vi "PLC.IO.vi"(7 "Idx":i32, 8 "error in":errorcluster, 10 "DbRun":bool, 11 "Data_in":T1={"Status"={"Idx"=0, "ConnRef"=0, "State"=enum."Off", "LiveBitTimer"=timestamp(0 s since 1904-01-01)}, "Sets"={"Enable"=FALSE, "IP"="", "Rack"=0, "Slot"=0, "LifeBitTimer_s"=0.0, "DataBlockAddr_PCStatus"=0, "DataBlockAddr_PLCStatus"=1, "DataBlockAddr_PLCNewData"=[], "DataBlockSize_PLCNewData"=[], "DataBlockAddr_PLCChangeOver"=[], "DataBlockSize_PLCChangeOver"=[], "DataBlockAddr_PCChangeOver"=[], "DataBlockAddr_PLCCheckStatus"=[], "DataBlockSize_PLCCheckStatus"=[], "DataBlockAddr_PCCheckStatus"=[], "System"=""}, "PCstatus"={"General"={"LifeBit"=FALSE, "DbRun"=FALSE}, "Stations"=[]}, "PLCstatus"={"General"={"LifeBit"=FALSE}, "Stations"=[]}}) -> (0 "error out":errorcluster, 3 "Data_out":T1={"Status"={"Idx"=0, "ConnRef"=0, "State"=enum."Off", "LiveBitTimer"=timestamp(0 s since 1904-01-01)}, "Sets"={"Enable"=FALSE, "IP"="", "Rack"=0, "Slot"=0, "LifeBitTimer_s"=0.0, "DataBlockAddr_PCStatus"=0, "DataBlockAddr_PLCStatus"=1, "DataBlockAddr_PLCNewData"=[], "DataBlockSize_PLCNewData"=[], "DataBlockAddr_PLCChangeOver"=[], "DataBlockSize_PLCChangeOver"=[], "DataBlockAddr_PCChangeOver"=[], "DataBlockAddr_PLCCheckStatus"=[], "DataBlockSize_PLCCheckStatus"=[], "DataBlockAddr_PCCheckStatus"=[], "System"=""}, "PCstatus"={"General"={"LifeBit"=FALSE, "DbRun"=FALSE}, "Stations"=[]}, "PLCstatus"={"General"={"LifeBit"=FALSE}, "Stations"=[]}})   [LabVIEW 2016]
doc: "Read data block from PLC to PC and write data block from PC to PLC. Control live bit of PC\n\nWabco 2017 All right reserved\nAuthor: maciej.szupienko@wabco-auto.com"
uses:
  PLC.Data.ctl
  PLC.Data.Status.ctl
  PLC.State.ctl
  PLC.Data.Sets.ctl
  LowLevel/PLC.DataBlock.PCstatus.ctl
  LowLevel/PLC.DataBlock.PCstatus.General.ctl
  LowLevel/PLC.DataBlock.PCstatus.Station.ctl
  LowLevel/PLC.DataBlock.PLCstatus.ctl
  LowLevel/PLC.DataBlock.PLCstatus.General.ctl
  LowLevel/PLC.DataBlock.PLCstatus.Station.ctl
  tools/EventLog/EventLog.EventSource.ctl
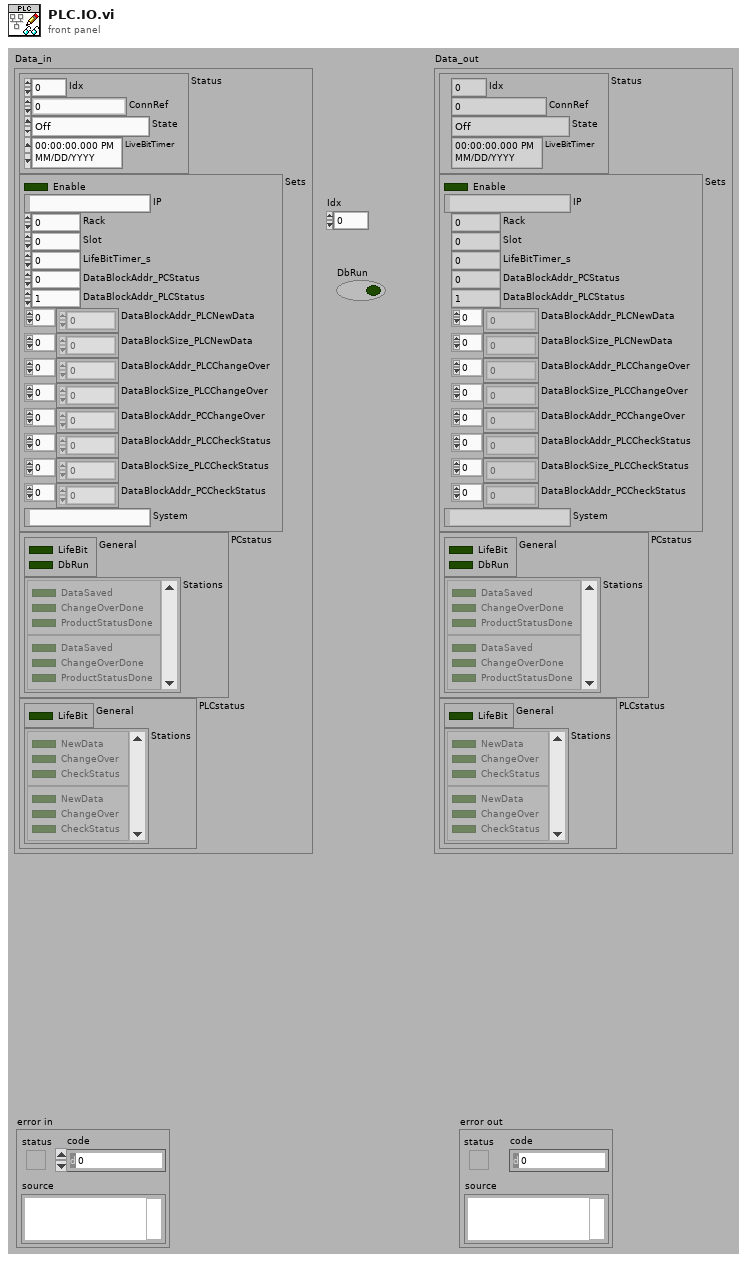
[diagram p1: front panel]
types:
  T1 = typedef "PLC.Data.ctl" = cluster{"Status":T2, "Sets":T4, "PCstatus":T5, "PLCstatus":T8}
  T2 = typedef "PLC.Data.Status.ctl" = cluster{"Idx":i32, "ConnRef":u64, "State":T3, "LiveBitTimer":timestamp}
  T3 = typedef "PLC.State.ctl" = enum32{"Off", "Error", "Idle", "Run"}
  T4 = typedef "PLC.Data.Sets.ctl" = cluster{"Enable":bool, "IP":string, "Rack":i32, "Slot":i32, "LifeBitTimer_s":dbl, "DataBlockAddr_PCStatus":i32, "DataBlockAddr_PLCStatus":i32, "DataBlockAddr_PLCNewData":i32[], "DataBlockSize_PLCNewData":i32[], "DataBlockAddr_PLCChangeOver":i32[], "DataBlockSize_PLCChangeOver":i32[], "DataBlockAddr_PCChangeOver":i32[], "DataBlockAddr_PLCCheckStatus":i32[], "DataBlockSize_PLCCheckStatus":i32[], "DataBlockAddr_PCCheckStatus":i32[], "System":string}
  T5 = typedef "PLC.DataBlock.PCstatus.ctl" = cluster{"General":T6, "Stations":T7[]}
  T6 = typedef "PLC.DataBlock.PCstatus.General.ctl" = cluster{"LifeBit":bool, "DbRun":bool}
  T7 = typedef "PLC.DataBlock.PCstatus.Station.ctl" = cluster{"DataSaved":bool, "ChangeOverDone":bool, "ProductStatusDone":bool}
  T8 = typedef "PLC.DataBlock.PLCstatus.ctl" = cluster{"General":T9, "Stations":T10[]}
  T9 = typedef "PLC.DataBlock.PLCstatus.General.ctl" = cluster{"LifeBit":bool}
  T10 = typedef "PLC.DataBlock.PLCstatus.Station.ctl" = cluster{"NewData":bool, "ChangeOver":bool, "CheckStatus":bool}
  T11 = typedef "EventLog.EventSource.ctl" = enum16{"All", "Gui", "Ref", "File", "Arch", "Seq", "CPX", "DB", "Laser", "Scan.P", "Scan.O", "PLC"}
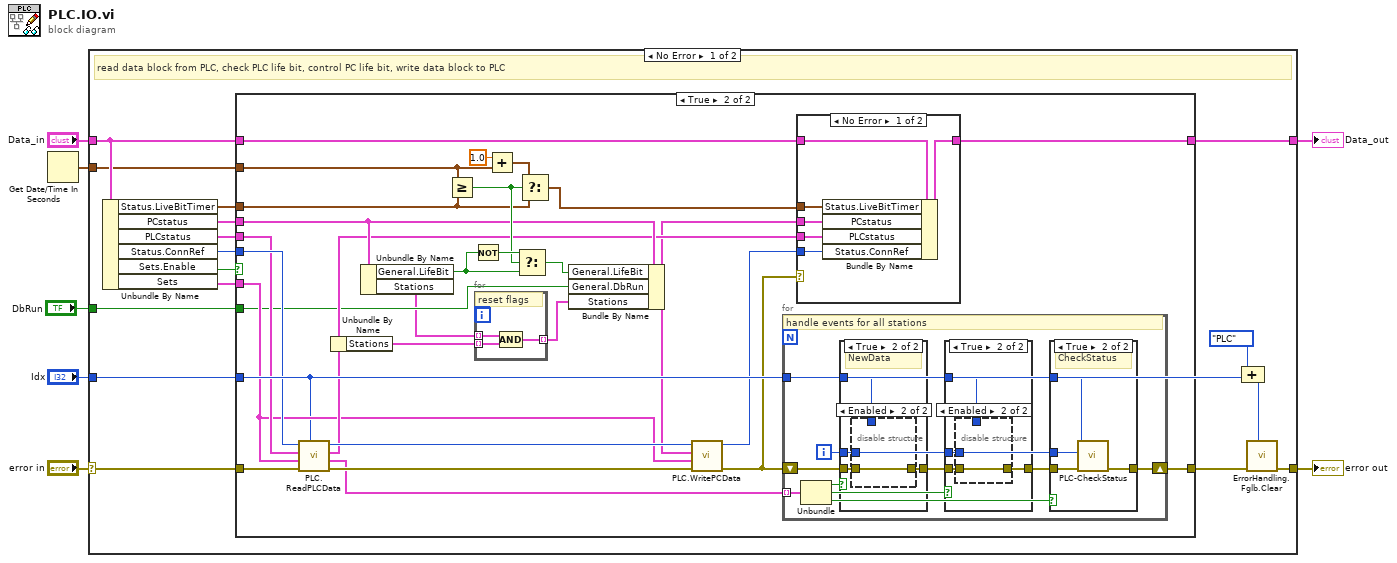
[diagram p0: block diagram]
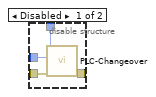
[diagram p5: hidden frame]
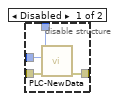
[diagram p7: hidden frame]
diagram:
  n1 = Get Date/Time In Seconds() -> (seconds since 1Jan1904=w3:timestamp)
  n2 = case shown="No Error" "error in" {
    selector: "error in" -> [w20 w101]
    tunnel: [w22 w101] -> w4
    tunnel: "Data_in" -> [w21 w100]
    tunnel: [w23 w100] -> w6
    tunnel: w3 -> [w19 _]
    tunnel: "Idx" -> [w11 _]
    tunnel: "DbRun" -> [w9 _]
    frame No Error {
      # "read data block from PLC, check PLC life bit, control PC life bit, write data block to PLC"
      n3 = Unbundle By Name(w21) -> ("Status.LiveBitTimer"=w18:timestamp, "PCstatus"=w17:T5, "PLCstatus"=w14:T8, "Status.ConnRef"=w16:u64, "Sets.Enable"=w13:bool, "Sets"=w12:T4)
      n4 = case shown="True" w13 {
        tunnel: [w25 w54] -> w23
        tunnel: w21 -> [w25 w53]
        tunnel: w20 -> [w24 w39]
        tunnel: w19 -> [_ w50]
        tunnel: w18 -> [_ w49]
        tunnel: w17 -> [_ w48]
        tunnel: w16 -> [_ w41]
        tunnel: [w24 w45] -> w15
        tunnel: w14 -> [_ w40]
        tunnel: w12 -> [_ w35]
        tunnel: w11 -> [_ w34]
        tunnel: w9 -> [_ w30]
        frame False {
        }
        frame True {
          n5 = call "PLC.ReadPLCData.vi"("Idx"=w34, "error in (no error)"=w39, "Sets"=w35, "PLCdata in"=w40, "Ref in"=w41) -> ("error out"=w36:errorcluster, "Events"=w31:T10[], "PLCdata out"=w37:T8, "Ref out"=w38:u64)  [unwired: 3 in]
          n6 = Unbundle By Name(w37) -> ("Stations"=w47:T10[])
          n7 = Unbundle By Name(w48) -> ("General.LifeBit"=w46:bool, "Stations"=w29:T7[])
          n8 = Greater Or Equal?(x=w50, y=w49) -> (x >= y?=w51:bool)
          n9 = Not(x=w46) -> (.not. x?=w52:bool)
          n10 = for {
            tunnel: w47 -> [w91] mode=indexing
            tunnel: w29 -> [w92] mode=indexing
            tunnel: [w90] -> w27 mode=indexing
            # "reset flags"
            n11 = Compound Arithmetic op=AND(w92, w91) -> (w90:T7)
          }
          n12 = Add(x=1.0 ("y"), y=w50) -> (x+y=w44:timestamp)
          n13 = Select(t=w52, s=w51, f=w46) -> (s? t:f=w26:bool)
          n14 = Select(t=w44, s=w51, f=w49) -> (s? t:f=w42:timestamp)
          n15 = Bundle By Name(cluster=w48, "General.LifeBit"=w26, "General.DbRun"=w30, "Stations"=w27) -> (w28:T5)
          n16 = call "PLC.WritePCData.vi"("error in (no error)"=w36, "Sets"=w35, "PCdata in"=w28, "Ref in"=w38) -> ("error out"=w32:errorcluster, "Ref out"=w33:u64)  [unwired: 5 in, 1 out]
          n17 = for {
            tunnel: w34 -> [w56]
            shift-right: [w55] -> w45
            shift-left: w32 -> [w64]
            tunnel: w31 -> [w63] mode=indexing
            i -> [w57]
            # "handle events for all stations"
            n18 = Unbundle(w63) -> ("NewData"=w62:bool, "ChangeOver"=w61:bool, "CheckStatus"=w58:bool)
            n19 = case shown="True" w62 {
              tunnel: w64 -> [w80 w84]
              tunnel: [w80 w83] -> w60
              tunnel: w56 -> [_ w82]
              tunnel: w57 -> [_ w81]
              frame False {
              }
              frame True {
                # "NewData"
                n20 = disable-structure shown="Enabled" {
                  disable-tunnel: w84 -> [w88 w89]
                  disable-tunnel: [w87 w89] -> w83
                  disable-tunnel: w82 -> [w86 _]
                  disable-tunnel: w81 -> [w85 _]
                  frame Disabled {
                    n21 = call "PLC-NewData.vi"("error in"=w88, "Slot"=w85, "Idx"=w86) -> ("error out"=w87:errorcluster)  [unwired: 8 in]
                  }
                  frame Enabled {
                  }
                }
              }
            }
            n22 = case shown="True" w61 {
              tunnel: w60 -> [w70 w71]
              tunnel: [w70 w74] -> w59
              tunnel: w56 -> [_ w73]
              tunnel: w57 -> [_ w72]
              frame False {
                # "ChangeOver"
              }
              frame True {
                n23 = disable-structure shown="Enabled" {
                  disable-tunnel: [w78 w79] -> w74
                  disable-tunnel: w73 -> [w77 _]
                  disable-tunnel: w72 -> [w76 _]
                  disable-tunnel: w71 -> [w75 w79]
                  frame Disabled {
                    n24 = call "PLC-Changeover.vi"("error in"=w75, "Slot"=w76, "Idx"=w77) -> ("error out"=w78:errorcluster)  [unwired: 8 in]
                  }
                  frame Enabled {
                  }
                }
              }
            }
            n25 = case shown="True" w58 {
              tunnel: w59 -> [w65 w66]
              tunnel: [w65 w69] -> w55
              tunnel: w56 -> [_ w68]
              tunnel: w57 -> [_ w67]
              frame False {
              }
              frame True {
                # "CheckStatus"
                n26 = call "PLC-CheckStatus.vi"("error in"=w66, "Slot"=w67, "Idx"=w68) -> ("error out"=w69:errorcluster)  [unwired: 8 in]
              }
            }
          }
          n27 = case shown="No Error" w32 {
            tunnel: [w98 w99] -> w54
            tunnel: w53 -> [w97 w99]
            tunnel: w28 -> [w96 _]
            tunnel: w37 -> [w95 _]
            tunnel: w42 -> [w94 _]
            tunnel: w33 -> [w93 _]
            frame No Error {
              n28 = Bundle By Name(cluster=w97, "Status.LiveBitTimer"=w94, "PCstatus"=w96, "PLCstatus"=w95, "Status.ConnRef"=w93) -> (w98:T1)
            }
            frame Error {
            }
          }
        }
      }
      n29 = Compound Arithmetic op=ADD(EventLog.EventSource."PLC" ("Event source"), w11) -> (w10:i32)
      n30 = call "ErrorHandling.Fglb.Clear.vi"("Event source"=w10, "error in (no error)"=w15) -> ("error out"=w22:errorcluster)  [unwired: 9 in]
    }
    frame Error {
    }
  }
  "error out" <- w4
  "Data_out" <- w6
